vi "Get Wheel Type.vi"(8 "error in (no error)":errorcluster, 11 "steering wheel in":refnum<class "NI_Robotics_Steering Wheel.lvclass">) -> (0 "error out":errorcluster, 2 "wheel type":string, 3 "steering wheel out":refnum<class "NI_Robotics_Steering Wheel.lvclass">)   [LabVIEW 2017, in "NI_Robotics_Steering Wheel.lvclass"]
uses:
  <vilib>/robotics/Steering/Steering Wheel/NI_Robotics_Steering Wheel.lvclass
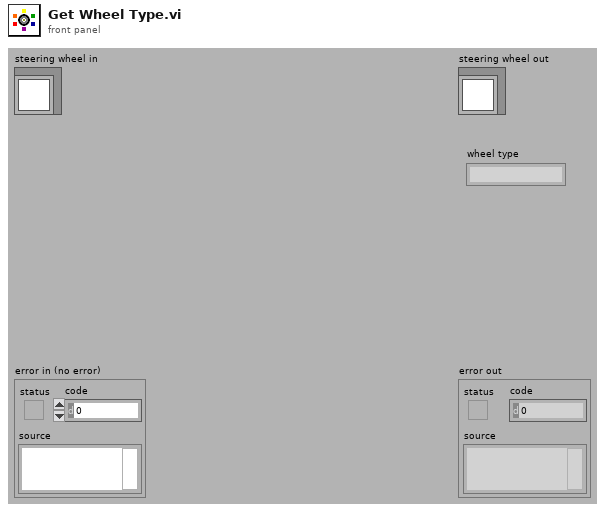
[diagram p1: front panel]
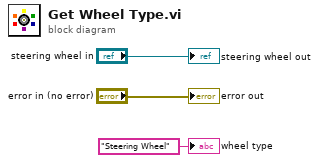
[diagram p0: block diagram]
diagram:
  "error out" <- "error in (no error)"
  "steering wheel out" <- "steering wheel in"
  "wheel type" <- "Steering Wheel" ("Wheel Type")
